vi "Check command.vi"(4 "error in (no error)":errorcluster, 6 "Is initialized":bool, 7 "Module mailbox":T1) -> (0 "error out":errorcluster, 1 "Command Data":variant, 2 "Command":T2)   [LabVIEW 2021, in "THz source modeule.lvlib"]
uses:
  THz source modeule.lvlib
  ctl/THz commands enum.ctl
  Messenger service/Data types/Mailbox address.ctl
  ctl/THz Message for module.ctl
  Messenger service/MessengerLib.lvlib
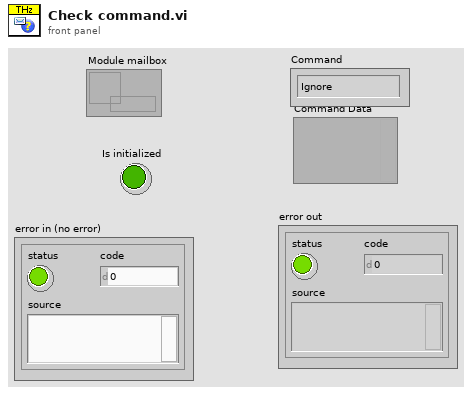
[diagram p1: front panel]
types:
  T1 = typedef "MessengerLib.lvlib/Mailbox address.ctl" = refnum<queue>
  T2 = typedef "THz source modeule.lvlib/THz commands enum.ctl" = enum16{"Ignore", "Initialize", "Update", "Set parameters", "Disconnect", "End"}
  T3 = typedef "THz source modeule.lvlib/THz Message for module.ctl" = cluster{"Command":T2, "Data":variant}
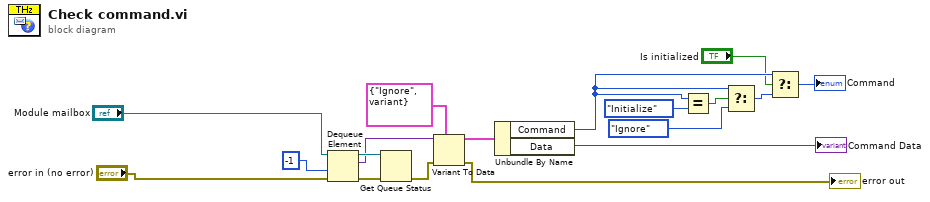
[diagram p0: block diagram]
diagram:
  n1 = Dequeue Element(queue="Module mailbox", timeout in ms (-1)=-1, error in (no error)="error in (no error)") -> (queue out=w4:T1, element=w3:variant, error out=w5:errorcluster)  [unwired: 1 out]
  n2 = Get Queue Status(queue=w4, error in (no error)=w5) -> (error out=w2:errorcluster)  [unwired: 1 in, 7 out]
  n3 = Variant To Data(error in=w2, type=T3 {"Command"=enum."Ignore", "Data"=variant} ("Msg for THz module"), Variant=w3) -> (data=w17:T3, error out=→"error out":errorcluster)
  n4 = Unbundle By Name(w17) -> ("Command"=w13:T2, "Data"=→"Command Data":variant)
  n5 = Equal?(x=w13, y=THz_commands_enum."Initialize" ("Command")) -> (x = y?=w14:bool)
  n6 = Select(t=w13, s=w14, f=THz_commands_enum."Ignore" ("Command")) -> (s? t:f=w15:T2)
  n7 = Select(t=w13, s="Is initialized", f=w15) -> (s? t:f=→"Command":T2)
